vi "Read Temperature control.vi"(11 "Test Framework in":refnum<class "Test Framework.lvclass">) -> (2 "Temperature control":T3, 3 "Test Framework out":refnum<class "Test Framework.lvclass">)   [LabVIEW 2020, in "Test Framework.lvclass"]
uses:
  Test Framework.lvclass
  Controls/Temperature and voltage array.ctl
  Controls/Temperature and voltage modes.ctl
  Test Framework.lvclass/Test Framework.ctl
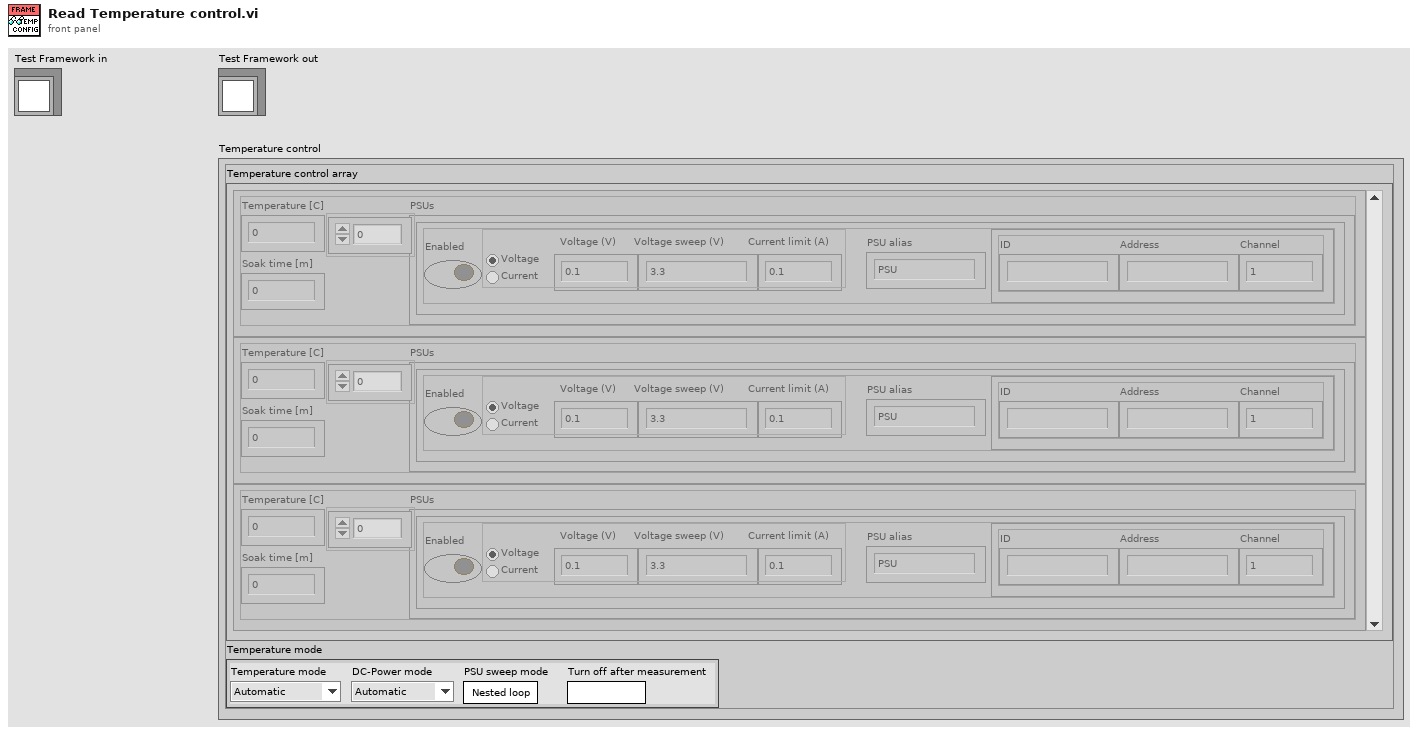
[diagram p1: front panel]
types:
  T1 = typedef "Test Framework.lvclass/Temperature and voltage array.ctl" = cluster{"Temperature [C]":dbl, "Soak time [m]":dbl, "PSUs":cluster{"Enabled":bool, "Source":enum32{"Voltage", "Current"}, "Drive (V/A)":dbl, "Sweep (V/A)":string, "Limit (A/V)":dbl, "PSU alias":string, "PSU info":cluster{"ID":string, "Address":string, "Channel":u8}}[]}[]
  T2 = typedef "Test Framework.lvclass/Temperature and voltage modes.ctl" = cluster{"Temperature mode":enum16{"Automatic", "Manual", "Off"}, "DC-Power mode":enum16{"Automatic", "Manual", "Off"}, "PSU sweep mode":bool, "Turn off after measurement":bool}
  T3 = cluster{"Temperature control array":T1, "Temperature mode":T2}
  T4 = cluster{"Environmental control array":T1, "Environmental mode":T2}
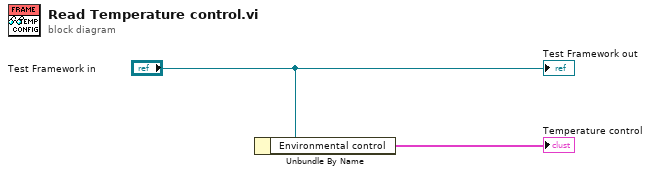
[diagram p0: block diagram]
diagram:
  n1 = Unbundle By Name("Test Framework in") -> ("Environmental control"=→"Temperature control":T4)
  "Test Framework out" <- "Test Framework in"
